vi "test IXX Writes to Source.vi"(8 "error in (no error)":errorcluster, 11 "TestCase in":refnum<class "Parameter Setting.lvclass">) -> (0 "error out":errorcluster, 3 "TestCase out":refnum<class "Parameter Setting.lvclass">)   [LabVIEW 2017, in "Static Errors Tests.lvlib" / "Parameter Setting.lvclass"]
uses:
  Parameter Setting.lvclass
  Parameter Setting.lvclass/Parameter Setting.ctl
  VIs/Write Numeric Scalar to Source (Base10 I64).vi
  VIs/Write Numeric Scalar to Source (Base10 I32).vi
  VIs/Write Numeric Scalar to Source (Base10 I16).vi
  VIs/Write Numeric Scalar to Source (Base10 I8).vi
  <vilib>/addons/_JKI Toolkits/VI Tester/TestCase.llb/TestCase.lvclass
  Static Errors.lvlib
  C:/Program Files (x86)/National Instruments/LabVIEW 2017/vi.lib/addons/_JKI Toolkits/VI Tester/TestCase.llb/TestCase.lvclass
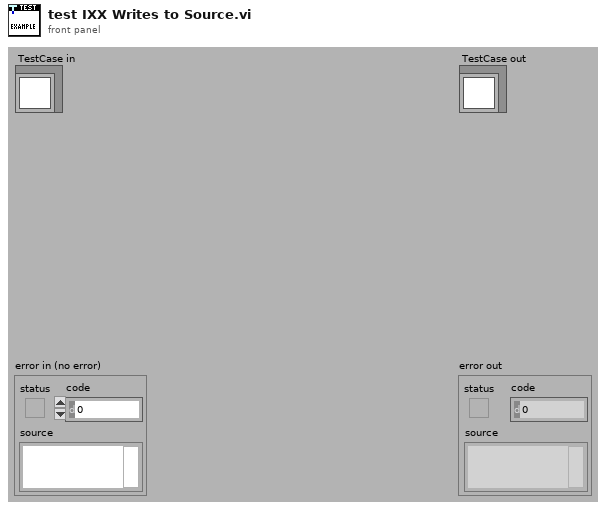
[diagram p1: front panel]
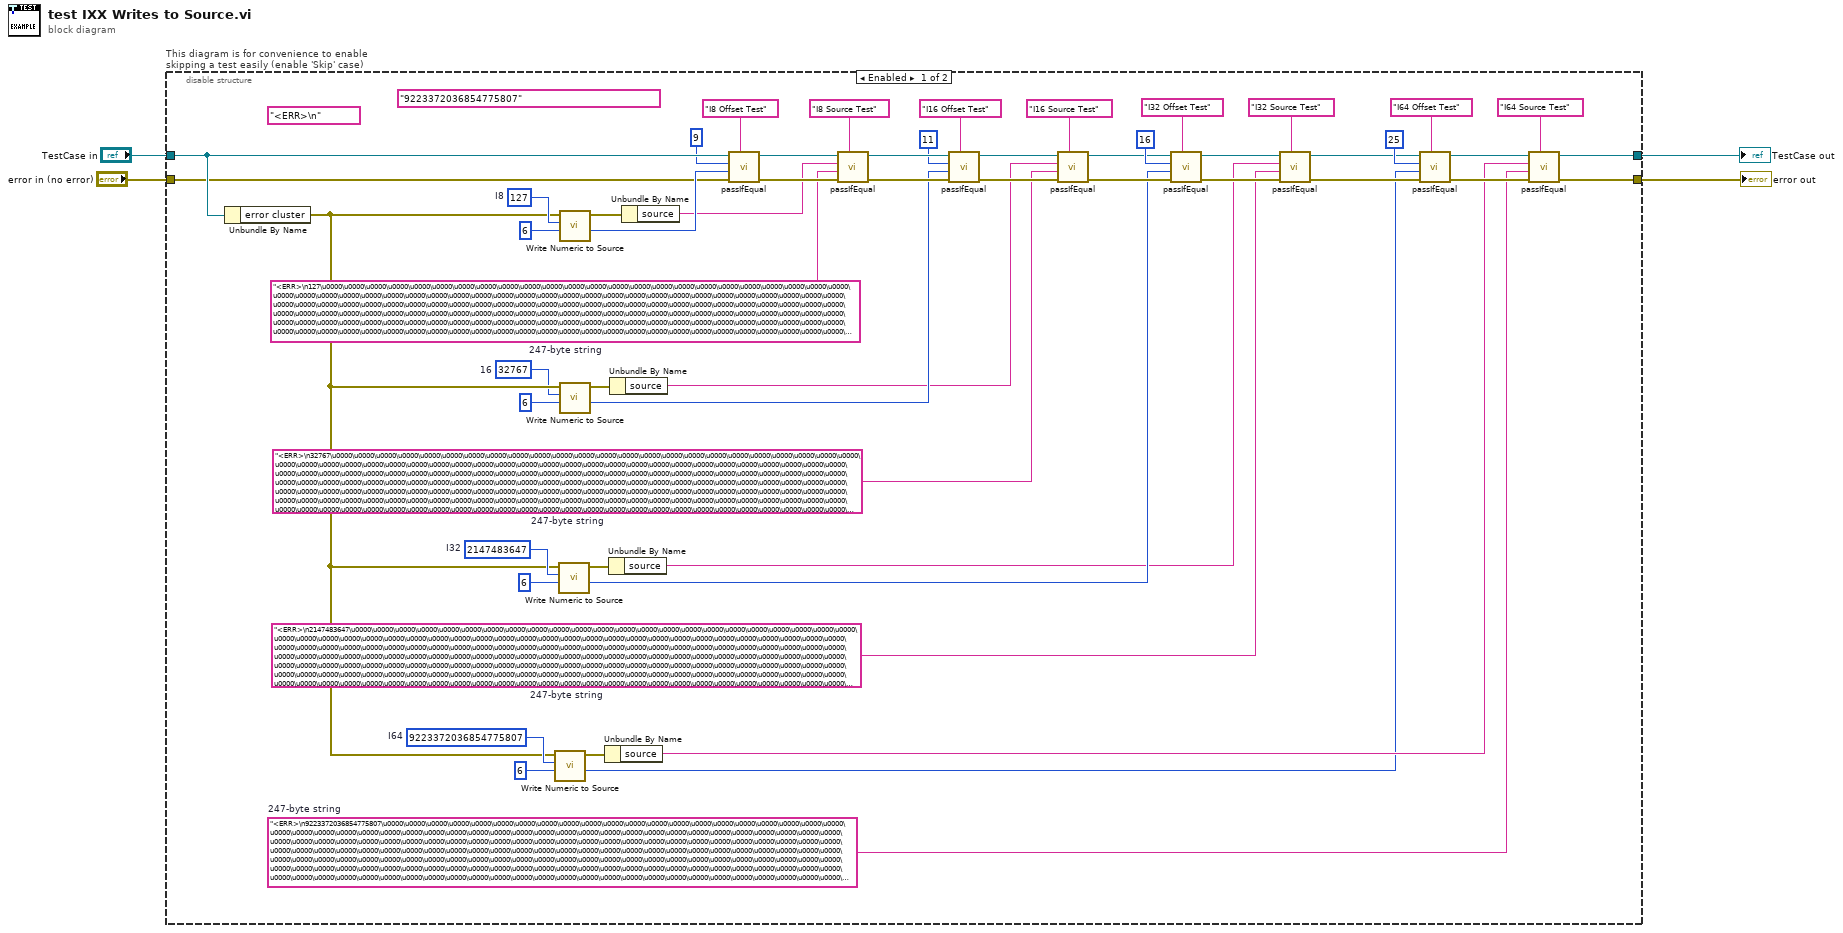
[diagram p0: block diagram]
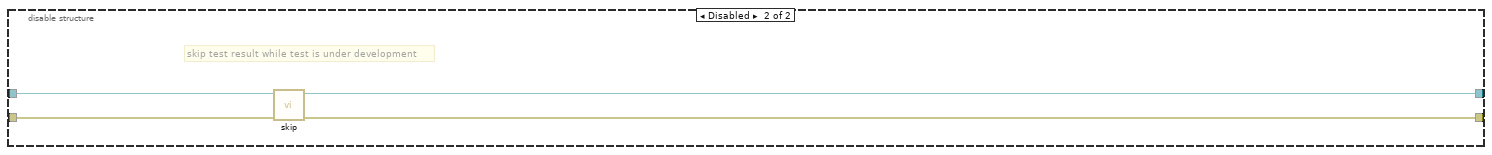
[diagram p2: hidden frame]
diagram:
  n1 = disable-structure "This diagram is for convenience to enable skipping a test easily (enable 'Skip' case)" shown="Enabled" {
    disable-tunnel: "TestCase in" -> [w55 w63]
    disable-tunnel: [w10 w61] -> w2
    disable-tunnel: [w9 w62] -> w1
    disable-tunnel: "error in (no error)" -> [w6 w60]
    frame Enabled {
      (unwired) "<ERR>\n"
      (unwired) "9223372036854775807"
      w23 = i64 9223372036854775807  # I64
      w12 = "<ERR>\n9223372036854775807\u0000\u0000\u0000\u0000\u0000\u0000\u0000\u0000\u0000\u0000\u0000\u0000\u0000\u0000\u0000\u0000\u0000\u0000\u0000\u0000\u0000\u0000\u0000\u0000\u0000\u0000\u0000\u0000\u0000\u0000\u0000\u0000\u0000\u0000\u0000\u0000\u0000\u0000\u0000\u0000\u0000\u0000\u0000\u0000\u0000\u0000\u0000\u0000\u0000\u0000\u0000\u0000\u0000\u0000\u0000\u0000\u0000\u0000\u0000\u0000\u0000\u0000\u0000\u0000\u0000\u0000\u0000\u0000\u0000\u0000\u0000\u0000\u0000\u0000\u0000\u0000\u0000\u0000\u0000\u0000\u0000\u0000\u0000\u0000\u0000\u0000\u0000\u0000\u0000\u0000\u0000\u0000\u0000\u0000\u0000\u0000\u0000\u0000\u0000\u0000\u0000\u0000\u0000\u0000\u0000\u0000\u0000\u0000\u0000\u0000\u0000\u0000\u0000\u0000\u0000\u0000\u0000\u0000\u0000\u0000\u0000\u0000\u0000\u0000\u0000\u0000\u0000\u0000\u0000\u0000\u0000\u0000\u0000\u0000\u0000\u0000\u0000\u0000\u0000\u0000\u0000\u0000\u0000\u0000\u0000\u0000\u0000\u0000\u0000\u0000\u0000\u0000\u0000\u0000\u0000\u0000\u0000\u0000\u0000\u0000\u0000\u0000\u0000\u0000\u0000\u0000\u0000\u0000\u0000\u0000\u0000\u0000\u0000\u0000\u0000\u0000\u0000\u0000\u0000\u0000\u0000\u0000\u0000\u0000\u0000\u0000\u0000\u0000\u0000\u0000\u0000\u0000\u0000\u0000\u0000\u0000\u0000\u0000\u0000\u0000\u0000\u0000\u0000\u0000\u0000\u0000\u0000\u0000\u0000\u0000\u0000\u0000\u0000\u0000\u0000\u0000\u0000\u0000\u0000\u0000\u0000\u0000"  # 247-byte string
      w36 = 2147483647  # I32
      w25 = "<ERR>\n2147483647\u0000\u0000\u0000\u0000\u0000\u0000\u0000\u0000\u0000\u0000\u0000\u0000\u0000\u0000\u0000\u0000\u0000\u0000\u0000\u0000\u0000\u0000\u0000\u0000\u0000\u0000\u0000\u0000\u0000\u0000\u0000\u0000\u0000\u0000\u0000\u0000\u0000\u0000\u0000\u0000\u0000\u0000\u0000\u0000\u0000\u0000\u0000\u0000\u0000\u0000\u0000\u0000\u0000\u0000\u0000\u0000\u0000\u0000\u0000\u0000\u0000\u0000\u0000\u0000\u0000\u0000\u0000\u0000\u0000\u0000\u0000\u0000\u0000\u0000\u0000\u0000\u0000\u0000\u0000\u0000\u0000\u0000\u0000\u0000\u0000\u0000\u0000\u0000\u0000\u0000\u0000\u0000\u0000\u0000\u0000\u0000\u0000\u0000\u0000\u0000\u0000\u0000\u0000\u0000\u0000\u0000\u0000\u0000\u0000\u0000\u0000\u0000\u0000\u0000\u0000\u0000\u0000\u0000\u0000\u0000\u0000\u0000\u0000\u0000\u0000\u0000\u0000\u0000\u0000\u0000\u0000\u0000\u0000\u0000\u0000\u0000\u0000\u0000\u0000\u0000\u0000\u0000\u0000\u0000\u0000\u0000\u0000\u0000\u0000\u0000\u0000\u0000\u0000\u0000\u0000\u0000\u0000\u0000\u0000\u0000\u0000\u0000\u0000\u0000\u0000\u0000\u0000\u0000\u0000\u0000\u0000\u0000\u0000\u0000\u0000\u0000\u0000\u0000\u0000\u0000\u0000\u0000\u0000\u0000\u0000\u0000\u0000\u0000\u0000\u0000\u0000\u0000\u0000\u0000\u0000\u0000\u0000\u0000\u0000\u0000\u0000\u0000\u0000\u0000\u0000\u0000\u0000\u0000\u0000\u0000\u0000\u0000\u0000\u0000\u0000\u0000\u0000\u0000\u0000\u0000\u0000\u0000\u0000\u0000\u0000\u0000\u0000\u0000\u0000\u0000\u0000"  # 247-byte string
      w7 = i16 32767  # 16
      w38 = "<ERR>\n32767\u0000\u0000\u0000\u0000\u0000\u0000\u0000\u0000\u0000\u0000\u0000\u0000\u0000\u0000\u0000\u0000\u0000\u0000\u0000\u0000\u0000\u0000\u0000\u0000\u0000\u0000\u0000\u0000\u0000\u0000\u0000\u0000\u0000\u0000\u0000\u0000\u0000\u0000\u0000\u0000\u0000\u0000\u0000\u0000\u0000\u0000\u0000\u0000\u0000\u0000\u0000\u0000\u0000\u0000\u0000\u0000\u0000\u0000\u0000\u0000\u0000\u0000\u0000\u0000\u0000\u0000\u0000\u0000\u0000\u0000\u0000\u0000\u0000\u0000\u0000\u0000\u0000\u0000\u0000\u0000\u0000\u0000\u0000\u0000\u0000\u0000\u0000\u0000\u0000\u0000\u0000\u0000\u0000\u0000\u0000\u0000\u0000\u0000\u0000\u0000\u0000\u0000\u0000\u0000\u0000\u0000\u0000\u0000\u0000\u0000\u0000\u0000\u0000\u0000\u0000\u0000\u0000\u0000\u0000\u0000\u0000\u0000\u0000\u0000\u0000\u0000\u0000\u0000\u0000\u0000\u0000\u0000\u0000\u0000\u0000\u0000\u0000\u0000\u0000\u0000\u0000\u0000\u0000\u0000\u0000\u0000\u0000\u0000\u0000\u0000\u0000\u0000\u0000\u0000\u0000\u0000\u0000\u0000\u0000\u0000\u0000\u0000\u0000\u0000\u0000\u0000\u0000\u0000\u0000\u0000\u0000\u0000\u0000\u0000\u0000\u0000\u0000\u0000\u0000\u0000\u0000\u0000\u0000\u0000\u0000\u0000\u0000\u0000\u0000\u0000\u0000\u0000\u0000\u0000\u0000\u0000\u0000\u0000\u0000\u0000\u0000\u0000\u0000\u0000\u0000\u0000\u0000\u0000\u0000\u0000\u0000\u0000\u0000\u0000\u0000\u0000\u0000\u0000\u0000\u0000\u0000\u0000\u0000\u0000\u0000\u0000\u0000\u0000\u0000\u0000\u0000\u0000\u0000\u0000\u0000\u0000"  # 247-byte string
      w8 = "<ERR>\n127\u0000\u0000\u0000\u0000\u0000\u0000\u0000\u0000\u0000\u0000\u0000\u0000\u0000\u0000\u0000\u0000\u0000\u0000\u0000\u0000\u0000\u0000\u0000\u0000\u0000\u0000\u0000\u0000\u0000\u0000\u0000\u0000\u0000\u0000\u0000\u0000\u0000\u0000\u0000\u0000\u0000\u0000\u0000\u0000\u0000\u0000\u0000\u0000\u0000\u0000\u0000\u0000\u0000\u0000\u0000\u0000\u0000\u0000\u0000\u0000\u0000\u0000\u0000\u0000\u0000\u0000\u0000\u0000\u0000\u0000\u0000\u0000\u0000\u0000\u0000\u0000\u0000\u0000\u0000\u0000\u0000\u0000\u0000\u0000\u0000\u0000\u0000\u0000\u0000\u0000\u0000\u0000\u0000\u0000\u0000\u0000\u0000\u0000\u0000\u0000\u0000\u0000\u0000\u0000\u0000\u0000\u0000\u0000\u0000\u0000\u0000\u0000\u0000\u0000\u0000\u0000\u0000\u0000\u0000\u0000\u0000\u0000\u0000\u0000\u0000\u0000\u0000\u0000\u0000\u0000\u0000\u0000\u0000\u0000\u0000\u0000\u0000\u0000\u0000\u0000\u0000\u0000\u0000\u0000\u0000\u0000\u0000\u0000\u0000\u0000\u0000\u0000\u0000\u0000\u0000\u0000\u0000\u0000\u0000\u0000\u0000\u0000\u0000\u0000\u0000\u0000\u0000\u0000\u0000\u0000\u0000\u0000\u0000\u0000\u0000\u0000\u0000\u0000\u0000\u0000\u0000\u0000\u0000\u0000\u0000\u0000\u0000\u0000\u0000\u0000\u0000\u0000\u0000\u0000\u0000\u0000\u0000\u0000\u0000\u0000\u0000\u0000\u0000\u0000\u0000\u0000\u0000\u0000\u0000\u0000\u0000\u0000\u0000\u0000\u0000\u0000\u0000\u0000\u0000\u0000\u0000\u0000\u0000\u0000\u0000\u0000\u0000\u0000\u0000\u0000\u0000\u0000\u0000\u0000\u0000\u0000\u0000\u0000"  # 247-byte string
      w59 = i8 127  # I8
      n2 = Unbundle By Name(w55) -> ("error cluster"=w21:errorcluster)
      n3 = call-poly "Write Numeric to Source.vi"("offset"=6, "value"=w23, "error in"=w21) -> ("new offset"=w11:i32, "error out"=w22:errorcluster)  [unwired: 7 in]
      n4 = call-poly "Write Numeric to Source.vi"("offset"=6, "value"=w36, "error in"=w21) -> ("new offset"=w27:i32, "error out"=w37:errorcluster)  [unwired: 7 in]
      n5 = call-poly "Write Numeric to Source.vi"("offset"=6, "value"=w59, "error in"=w21) -> ("new offset"=w54:i32, "error out"=w58:errorcluster)  [unwired: 7 in]
      n6 = call-poly "Write Numeric to Source.vi"("offset"=6, "value"=w7, "error in"=w21) -> ("new offset"=w43:i32, "error out"=w49:errorcluster)  [unwired: 7 in]
      n7 = Unbundle By Name(w22) -> ("source"=w13:string)
      n8 = Unbundle By Name(w37) -> ("source"=w26:string)
      n9 = Unbundle By Name(w49) -> ("source"=w39:string)
      n10 = Unbundle By Name(w58) -> ("source"=w44:string)
      n11 = call-dynamic "passIfEqual.vi"("custom report message (\"\")"="I8 Offset Test" ("custom report message (\"\")"), "error in (no error)"=w6, "y"=w54, "x"=9 ("offset"), "TestCase in"=w55) -> ("error out"=w56:errorcluster, "TestCase out"=w57:refnum<class "Parameter Setting.lvclass">)  [unwired: 5 in]
      n12 = call-dynamic "passIfEqual.vi"("custom report message (\"\")"="I8 Source Test" ("custom report message (\"\")"), "error in (no error)"=w56, "y"=w8, "x"=w44, "TestCase in"=w57) -> ("error out"=w46:errorcluster, "TestCase out"=w48:refnum<class "Parameter Setting.lvclass">)  [unwired: 5 in]
      n13 = call-dynamic "passIfEqual.vi"("custom report message (\"\")"="I16 Offset Test" ("custom report message (\"\")"), "error in (no error)"=w46, "y"=w43, "x"=11 ("offset"), "TestCase in"=w48) -> ("error out"=w45:errorcluster, "TestCase out"=w47:refnum<class "Parameter Setting.lvclass">)  [unwired: 5 in]
      n14 = call-dynamic "passIfEqual.vi"("custom report message (\"\")"="I16 Source Test" ("custom report message (\"\")"), "error in (no error)"=w45, "y"=w38, "x"=w39, "TestCase in"=w47) -> ("error out"=w28:errorcluster, "TestCase out"=w29:refnum<class "Parameter Setting.lvclass">)  [unwired: 5 in]
      n15 = call-dynamic "passIfEqual.vi"("custom report message (\"\")"="I32 Offset Test" ("custom report message (\"\")"), "error in (no error)"=w28, "y"=w27, "x"=16 ("offset"), "TestCase in"=w29) -> ("error out"=w31:errorcluster, "TestCase out"=w30:refnum<class "Parameter Setting.lvclass">)  [unwired: 5 in]
      n16 = call-dynamic "passIfEqual.vi"("custom report message (\"\")"="I32 Source Test" ("custom report message (\"\")"), "error in (no error)"=w31, "y"=w25, "x"=w26, "TestCase in"=w30) -> ("error out"=w15:errorcluster, "TestCase out"=w16:refnum<class "Parameter Setting.lvclass">)  [unwired: 5 in]
      n17 = call-dynamic "passIfEqual.vi"("custom report message (\"\")"="I64 Offset Test" ("custom report message (\"\")"), "error in (no error)"=w15, "y"=w11, "x"=25 ("offset"), "TestCase in"=w16) -> ("error out"=w14:errorcluster, "TestCase out"=w20:refnum<class "Parameter Setting.lvclass">)  [unwired: 5 in]
      n18 = call-dynamic "passIfEqual.vi"("custom report message (\"\")"="I64 Source Test" ("custom report message (\"\")"), "error in (no error)"=w14, "y"=w12, "x"=w13, "TestCase in"=w20) -> ("error out"=w9:errorcluster, "TestCase out"=w10:refnum<class "Parameter Setting.lvclass">)  [unwired: 5 in]
    }
    frame Disabled {
      # "skip test result while test is under development"
      n19 = call <vilib>:"skip.vi"("error in (no error)"=w60, "TestCase in"=w63) -> ("error out"=w62:errorcluster, "TestCase out"=w61:refnum<class "Parameter Setting.lvclass">)  [unwired: 8 in]
    }
  }
  "error out" <- w1
  "TestCase out" <- w2
